vi "programa4.vi"() -> ()   [LabVIEW 2011]
panel:
  out "Rango":string
  out "121-180":bool
  out "81-120":bool
  out "1-80":bool
  out "Velocidad":dbl(knob) scale=0.0..180.0
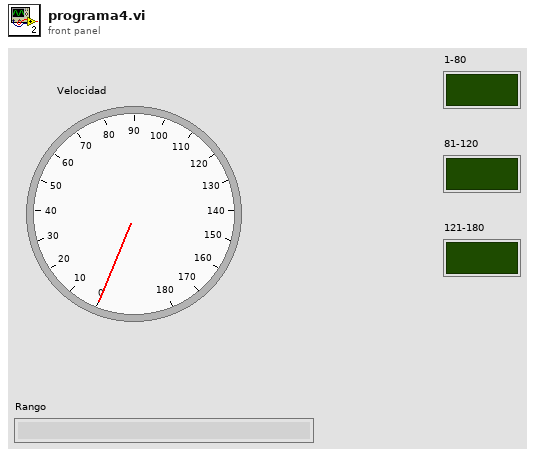
[diagram p1: front panel]
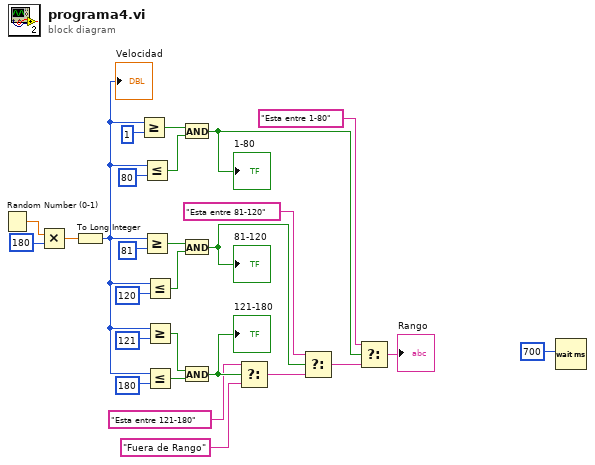
[diagram p0: block diagram]
diagram:
  n1 = Random Number (0-1)() -> (number: 0 to 1=w27:dbl)
  n2 = Multiply(x=w27, y=180) -> (x*y=w25:dbl)
  n3 = To Long Integer(number=w25) -> (32bit integer=w16:i32)
  "Velocidad" <- w16
  n4 = Greater Or Equal?(x=w16, y=1) -> (x >= y?=w22:bool)
  n5 = Less Or Equal?(x=w16, y=80) -> (x <= y?=w21:bool)
  n6 = Greater Or Equal?(x=w16, y=81) -> (x >= y?=w15:bool)
  n7 = Less Or Equal?(x=w16, y=120) -> (x <= y?=w14:bool)
  n8 = Greater Or Equal?(x=w16, y=121) -> (x >= y?=w13:bool)
  n9 = Less Or Equal?(x=w16, y=180) -> (x <= y?=w12:bool)
  n10 = And(x=w22, y=w21) -> (x .and. y?=w11:bool)
  "1-80" <- w11
  n11 = And(x=w15, y=w14) -> (x .and. y?=w8:bool)
  "81-120" <- w8
  n12 = And(x=w13, y=w12) -> (x .and. y?=w5:bool)
  "121-180" <- w5
  n13 = Select(t="Esta entre 121-180", s=w5, f="Fuera de Rango") -> (s? t:f=w3:string)
  n14 = Select(t="Esta entre 81-120", s=w8, f=w3) -> (s? t:f=w6:string)
  n15 = Select(t="Esta entre 1-80", s=w11, f=w6) -> (s? t:f=→"Rango":string)
  n16 = Wait (ms)(milliseconds to wait=700) -> ()  [unwired: 1 out]
